vi "StickyButton2.vi"(1 "Reset":bool, 2 "Time threshold (ms)":u32, 3 "Button Input":bool) -> (0 "Sticky Button":bool)   [LabVIEW 2020]
doc: "The input stays true for a certain number of seconds after release and it starts as false. The Time Threshold is the amount of time the output stays true after the input is released. This VI can be used as a debounce circuit or to keep a certain robot action active (e.g., a pre-spin of shooter wheels)."
uses:
  d4953c67-f53d-41fa-97a7-851cc2dfed5b.vi
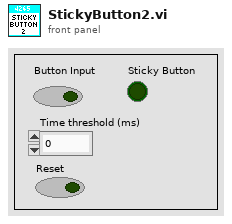
[diagram p1: front panel]
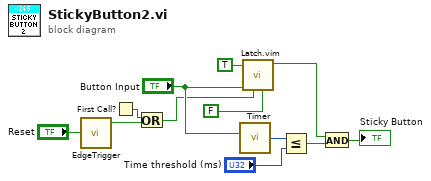
[diagram p0: block diagram]
diagram:
  n1 = call "EdgeTrigger.vi"("Input Signal"="Reset") -> ("Rising Edge Trigger"=w1:bool)  [unwired: 2 out]
  n2 = First Call?() -> (First Call?: T/F=w4:bool)
  n3 = Or(x=w4, y=w1) -> (x .or. y?=w3:bool)
  n4 = call "Timer.vi"("Reset Timer"="Button Input") -> ("Time (ms)"=w12:u32)
  n5 = call "Latch.vim"("Default Value"=FALSE, "Reset"=w3, "Latch Signal"="Button Input", "Latch Value"=TRUE) -> ("Latched"=w8:bool)  [unwired: 7 in]
  n6 = Less Or Equal?(x=w12, y="Time threshold (ms)") -> (x <= y?=w9:bool)
  n7 = And(x=w8, y=w9) -> (x .and. y?=→"Sticky Button":bool)
